vi "SWERVE_SIM_MODULE_CO_FGV.vi"(9 "in SwerveModuleMotorDmd":T1 {"SwerveMotorDmd" format="%17.4f"; "WheelMotorDmd" format="%17.4f"}, 10 "Index":i32, 11 "WRITE":bool) -> (3 "out SwerveModuleMotorDmd":T1 {"SwerveMotorDmd" format="%17.4f"; "WheelMotorDmd" format="%17.4f"})   [LabVIEW 2019]
uses:
  SWERVE_MODULE_MOTOR_CO.ctl
panel:
  # "This is purposefully \n\nNOT re-entrant."
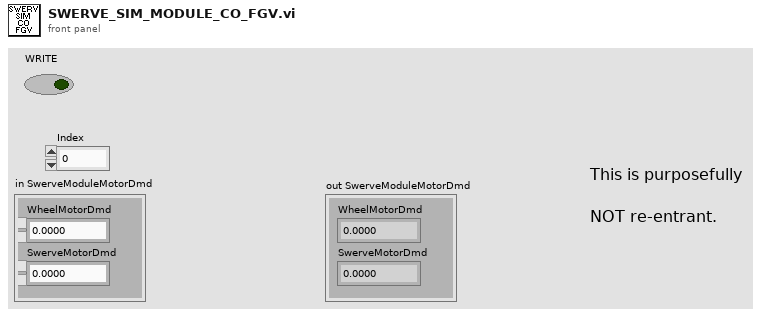
[diagram p1: front panel]
types:
  T1 = typedef "SWERVE_MODULE_MOTOR_CO.ctl" = cluster{"WheelMotorDmd":dbl, "SwerveMotorDmd":dbl}
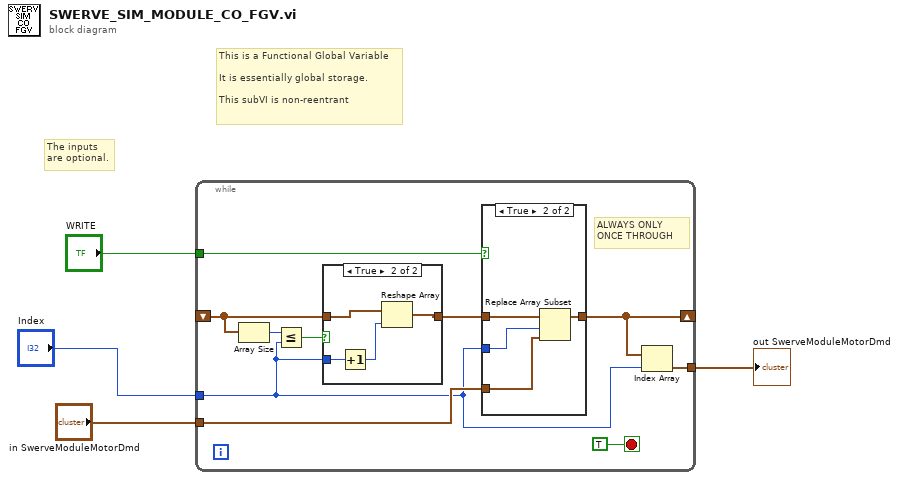
[diagram p0: block diagram]
diagram:
  # "The inputs \nare optional."
  # "This is a Functional Global Variable\n\nIt is essentially global storage.\n\nThis subVI is non-reentrant"
  n1 = while {
    shift-right: [w10] -> _
    shift-left: _ -> [w7]
    tunnel: "WRITE" -> [w13]
    tunnel: "in SwerveModuleMotorDmd" -> [w12]
    tunnel: "Index" -> [w5]
    tunnel: [w11] -> w1
    stop <- TRUE stop-if-true
    # "ALWAYS ONLY\nONCE THROUGH"
    n2 = Array Size(array=w7) -> (size(s)=w9:i32)
    n3 = Less Or Equal?(x=w9, y=w5) -> (x <= y?=w8:bool)
    n4 = case shown="True" w8 {
      tunnel: w7 -> [w15 w18]
      tunnel: [w15 w19] -> w6
      tunnel: w5 -> [_ w17]
      frame False {
      }
      frame True {
        n5 = Increment(x=w17) -> (x+1=w16:i32)
        n6 = Reshape Array(w18, w16) -> (w19:T1[])
      }
    }
    n7 = case shown="True" w13 {
      tunnel: [w20 w23] -> w10
      tunnel: w12 -> [_ w21]
      tunnel: w6 -> [w20 w22]
      tunnel: w5 -> [_ w24]
      frame False {
      }
      frame True {
        n8 = Replace Array Subset(array=w22, new element=w21, index=w24) -> (w23:T1[])
      }
    }
    n9 = Index Array(array=w10, index=w5) -> (element=w11:T1)
  }
  "out SwerveModuleMotorDmd" <- w1
